vi "Pico Status Code to Error Cluster.vi"(2 "error in":errorcluster, 3 "PICO_STATUS":u32) -> (0 "error out":errorcluster)   [LabVIEW 2016, in "pl1000.lvlib"]
uses:
  pl1000.lvlib
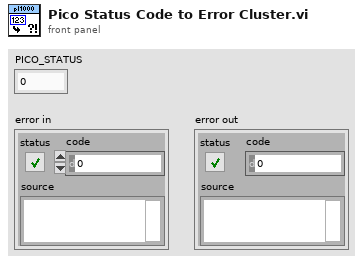
[diagram p1: front panel]
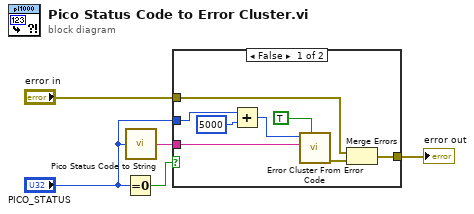
[diagram p0: block diagram]
diagram:
  n1 = Equal To 0?(x="PICO_STATUS") -> (x = 0?=w5:bool)
  n2 = call "Pico Status Code to String.vi"("PICO_STATUS"="PICO_STATUS") -> ("PICO_STATUS"=w4:string)
  n3 = case shown="False" w5 {
    tunnel: w4 -> [w12 _]
    tunnel: "error in" -> [w9 w14]
    tunnel: [w8 w14] -> w2
    tunnel: "PICO_STATUS" -> [w6 _]
    frame False {
      n4 = Add(x=w6, y=5000 ("error code (0)")) -> (x+y=w7:u32)
      n5 = call <vilib>:"Error Cluster From Error Code.vi"("show call chain? (False)"=TRUE, "error message (\"\")"=w12, "error code (0)"=w7) -> ("error out"=w10:errorcluster)  [unwired: 6 in]
      n6 = Merge Errors(w9, w10) -> (w8:errorcluster)
    }
    frame True {
    }
  }
  "error out" <- w2
